vi "Trilinear - Interpolation.vi"(8 "error in (no error)":errorcluster, 9 "XYZ Point":cluster{"X":dbl, "Y":dbl, "Z":dbl} {"Z" scale=0.01..10.0; "Y" scale=0.01..10.0; "X" scale=0.0..2.0}, 10 "Axis Vectors":T1, 11 "Values":dbl[][][](array[numeric])) -> (0 "error out":errorcluster, 3 "Interpolated Value":dbl)   [LabVIEW 2019]
uses:
  <vilib>/Analysis/Matrix/Datatypes/RealMatrix.ctl
  <vilib>/Analysis/7linalg.llb/Solve Linear Equations (single right hand).vi
  <vilib>/Analysis/baseanly.llb/Solve Linear Equations By Cholesky.vi
  <vilib>/Analysis/baseanly.llb/Real Matrix to Compact Array.vi
  <vilib>/Analysis/baseanly.llb/Real Compact Tri-Matrix Linear Eqs.vi
  <vilib>/Analysis/7linalg.llb/Solve Linear Eqs (General).vi
  <vilib>/Analysis/7linalg.llb/Solve Linear Eqs (Gen, single right hand).vi
  <vilib>/Analysis/NI_AALPro.lvlib
  <vilib>/Analysis/Matrix/NI_Matrix.lvlib
panel:
  out "Waveform Chart":dbl(graph)
  out "Bounding Axis - Indexes":i32[][](array[numeric])
  out "Bounding Axis - Values":dbl[][](array[numeric])
  out "Solution Vector":dbl[](array[numeric])
  out "Input Matrix":T2
  out "Known Vector":dbl[](array[numeric])
  # "Intermediate Calculations"
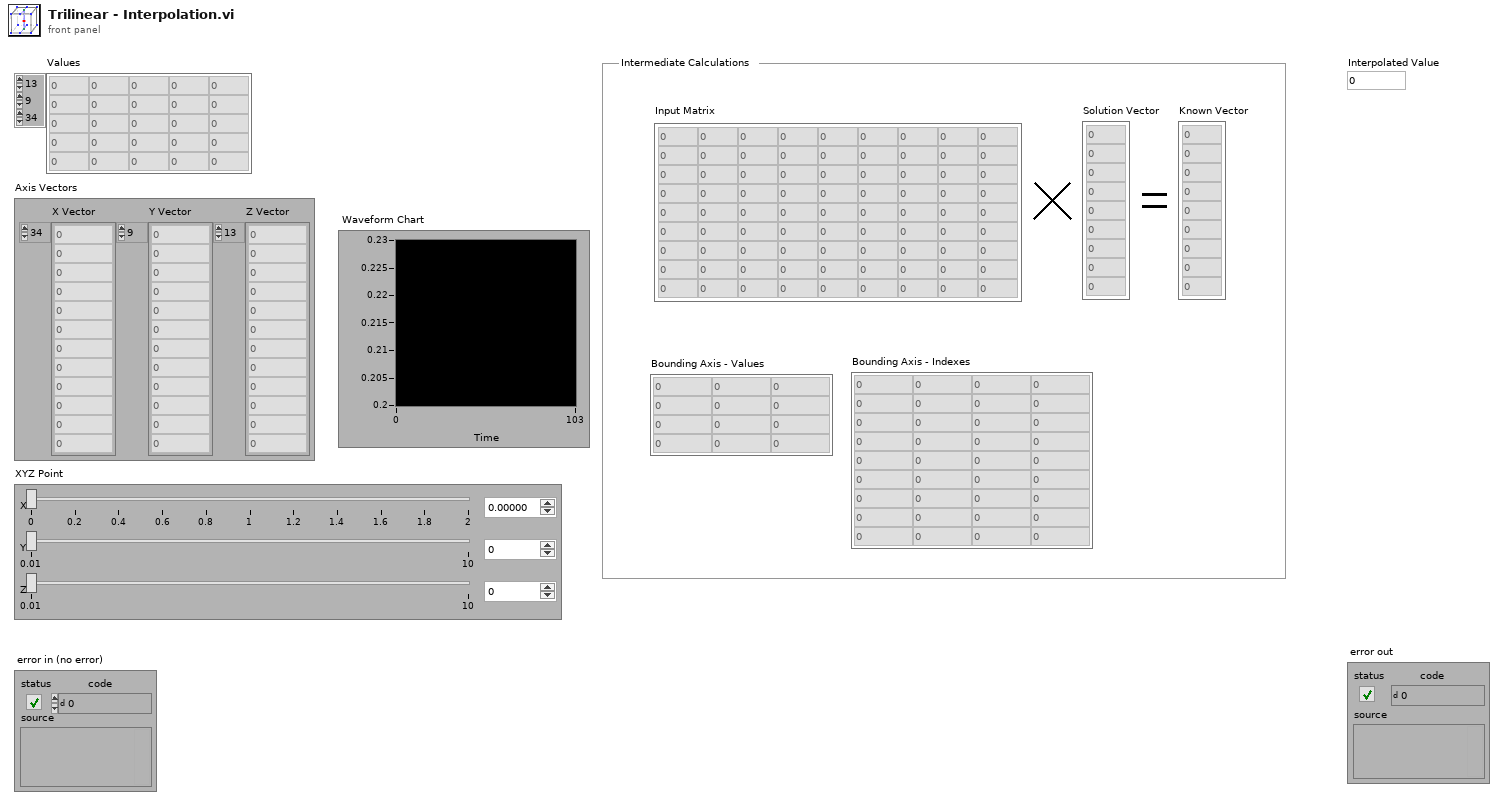
[diagram p1: front panel]
types:
  T1 = cluster{"X Vector":dbl[], "Y Vector":dbl[], "Z Vector":dbl[]}
  T2 = typedef "NI_Matrix.lvlib/RealMatrix.ctl" = dbl[][]
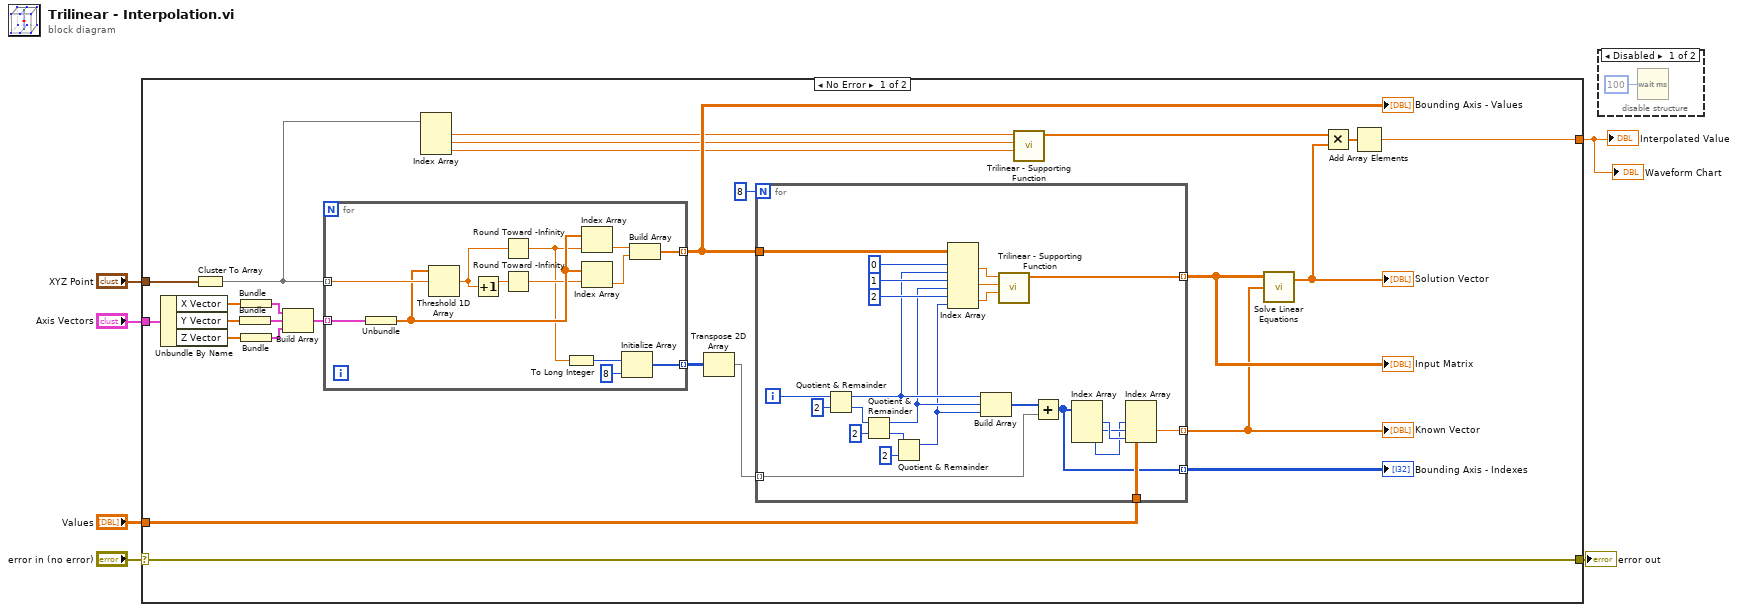
[diagram p0: block diagram]
diagram:
  n1 = case shown="No Error" "error in (no error)" {
    selector: "error in (no error)" -> [w20 w71]
    tunnel: "XYZ Point" -> [w29 _]
    tunnel: "Axis Vectors" -> [w24 _]
    tunnel: [w20 w71] -> w3
    tunnel: [w12 _] -> w1
    tunnel: "Values" -> [w9 _]
    frame No Error {
      n2 = Unbundle By Name(w24) -> ("X Vector"=w23:dbl[], "Y Vector"=w22:dbl[], "Z Vector"=w21:dbl[])
      n3 = Cluster To Array(cluster=w29) -> (array=w19:dbl[])
      n4 = Bundle("Y Vector"=w22) -> (w31:cluster{"Y Vector":dbl[]})  [unwired: 1 in]
      n5 = Bundle("X Vector"=w23) -> (w30:cluster{"X Vector":dbl[]})  [unwired: 1 in]
      n6 = Bundle("Z Vector"=w21) -> (w32:cluster{"Z Vector":dbl[]})  [unwired: 1 in]
      n7 = Build Array(w30, w31, w32) -> (w28:cluster{"Z Vector":dbl[]}[])
      n8 = for {
        tunnel: w19 -> [w69] mode=indexing
        tunnel: w28 -> [w70] mode=indexing
        tunnel: [w64] -> w26 mode=indexing
        tunnel: [w61] -> w11 mode=indexing
        n9 = Unbundle(w70) -> ("Z Vector"=w67:dbl[])
        n10 = Threshold 1D Array(2:w69, 3:w67) -> (0:w68:dbl)  [unwired: 1 in]
        n11 = Increment(x=w68) -> (x+1=w58:dbl)
        n12 = Round Toward -Infinity(1:w68) -> (0:w60:dbl)
        n13 = Round Toward -Infinity(1:w58) -> (0:w63:dbl)
        n14 = To Long Integer(number=w60) -> (32bit integer=w59:i32)
        n15 = Index Array(array=w67, index=w60) -> (element=w66:dbl)
        n16 = Index Array(array=w67, index=w63) -> (element=w65:dbl)
        n17 = Initialize Array(w59, 8 ("dimension size")) -> (w61:i32[])
        n18 = Build Array(w66, w65) -> (w64:dbl[])
      }
      "Bounding Axis - Values" <- w26
      n19 = Index Array(array=w19) -> (element #1=w18:dbl, element #2=w16:dbl, element #3=w17:dbl)  [unwired: 3 in]
      n20 = Transpose 2D Array(2D array=w11) -> (transposed array=w10:i32[][])
      n21 = for {
        N: 8 -> [_]
        tunnel: [w57] -> w25 mode=indexing
        tunnel: w26 -> [w54]
        tunnel: w10 -> [w39] mode=indexing
        tunnel: w9 -> [w38]
        tunnel: [w37] -> w8 mode=indexing
        tunnel: [w36] -> w7 mode=indexing
        i -> [w56]
        n22 = Quotient & Remainder(x=w56, y=2) -> (x-y*floor(x/y)=w43:i32, floor(x/y)=w51:i32)
        n23 = Quotient & Remainder(x=w51, y=2) -> (x-y*floor(x/y)=w42:i32, floor(x/y)=w47:i32)
        n24 = Quotient & Remainder(x=w47, y=2) -> (x-y*floor(x/y)=w41:i32)  [unwired: 1 out]
        n25 = Index Array(array=w54, index (row) #1=0 ("disabled index (row)"), index (col) #1=w43, index (row) #2=1 ("disabled index (row)"), index (col) #2=w42, index (row) #3=2 ("disabled index (row)"), index (col) #3=w41) -> (element #1=w46:dbl, element #2=w45:dbl, element #3=w44:dbl)
        n26 = Build Array(w43, w42, w41) -> (w40:i32[])
        n27 = call "Trilinear - Supporting Function.vi"("Z"=w44, "Y"=w45, "X"=w46) -> ("C Array"=w57:dbl[])  [unwired: 8 in]
        n28 = Add(x=w40, y=w39) -> (x+y=w36:i32[])
        n29 = Index Array(array=w36) -> (element #1=w35:i32, element #2=w34:i32, element #3=w33:i32)  [unwired: 3 in]
        n30 = Index Array(array=w38, index (dim 0)=w33, index (dim 1)=w34, index (dim 2)=w35) -> (element=w37:dbl)
      }
      "Known Vector" <- w8
      "Input Matrix" <- w25
      "Bounding Axis - Indexes" <- w7
      n31 = call "Trilinear - Supporting Function.vi"("Z"=w17, "Y"=w16, "X"=w18) -> ("C Array"=w14:dbl[])  [unwired: 8 in]
      n32 = call-poly <vilib>:"Solve Linear Equations.vi"("Known Vector"=w8, "Input Matrix"=w25) -> ("Solution Vector"=w15:dbl[])  [unwired: 1 in, 1 out]
      "Solution Vector" <- w15
      n33 = Multiply(x=w14, y=w15) -> (x*y=w13:dbl[])
      n34 = Add Array Elements(numeric array=w13) -> (sum=w12:dbl)
    }
    frame Error {
    }
  }
  "error out" <- w3
  "Interpolated Value" <- w1
  "Waveform Chart" <- w1
  n35 = disable-structure shown="Disabled" {
    frame Disabled {
      n36 = Wait (ms)(milliseconds to wait=u32 100) -> ()  [unwired: 1 out]
    }
    frame Enabled {
    }
  }
